vi "Write Frame History Depth.vi"(8 "error in (no error)":errorcluster, 10 "Frame History Depth":i32, 11 "Video Processor in":refnum<class "Video Processor.lvclass">) -> (0 "error out":errorcluster, 3 "Video Processor out":refnum<class "Video Processor.lvclass">)   [LabVIEW 2018, in "Video Processor.lvclass"]
uses:
  Video Processor.lvclass
  Video Processor.lvclass/Video Processor.ctl
  b3bbf2d5-da6e-4050-8ea6-dccdc7c034c8.vi
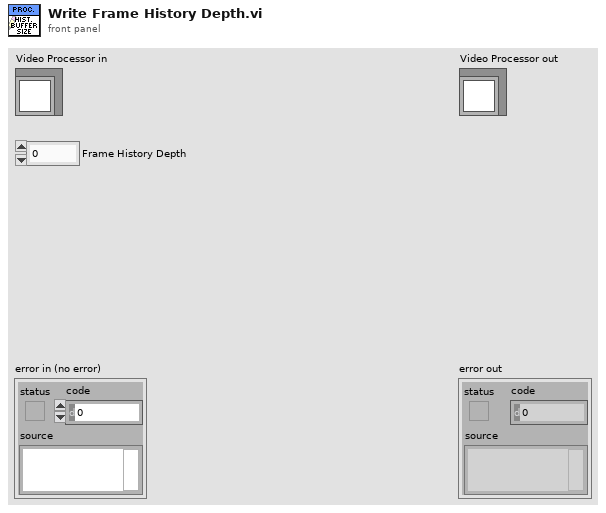
[diagram p1: front panel]
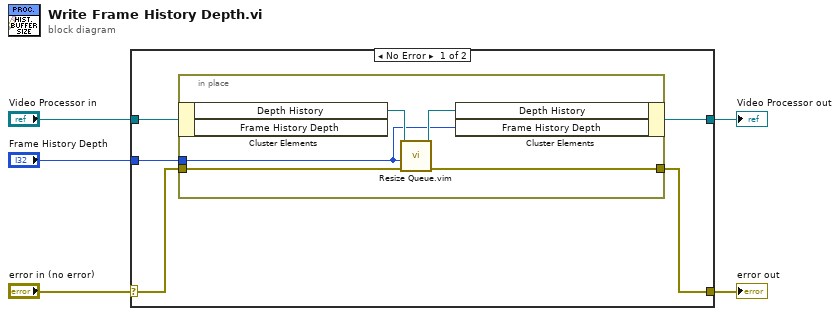
[diagram p0: block diagram]
diagram:
  n1 = case shown="No Error" "error in (no error)" {
    selector: "error in (no error)" -> [w7 w16]
    tunnel: [w6 w16] -> w4
    tunnel: [w9 w17] -> w2
    tunnel: "Video Processor in" -> [w10 w17]
    tunnel: "Frame History Depth" -> [w8 _]
    frame No Error {
      n2 = in-place {
        in-place-border: w7 -> [w14]
        in-place-border: w8 -> [w12]
        in-place-border: [w11] -> w6
        n3 = in-place-cluster #1(w10) -> ("Depth History"=w15:refnum<queue>)  [unwired: 1 out]
        n4 = call "Resize Queue.vim"("error in (no error)"=w14, "Size"=w12, "Queue In"=w15) -> ("error out"=w11:errorcluster, "Queue Out"=w13:refnum<queue>)  [unwired: 6 in, 1 out]
        n5 = in-place-cluster #1("Depth History"=w13, "Frame History Depth"=w12) -> (w9:refnum<class "Video Processor.lvclass">)
      }
    }
    frame Error {
    }
  }
  "error out" <- w4
  "Video Processor out" <- w2
